vi "ProcessBotMove.vi"(7 "MatchState":T1, 8 "error in (no error)":errorcluster, 9 "GameState":T2, 10 "BotPosition":T3, 11 "Bot in":T4) -> (0 "error out":errorcluster, 2 "NewPlayerPosition":T3, 3 "Bot out":T4)   [LabVIEW 2015, in "TronviewGame.lvlib" / "Game.lvclass"]
uses:
  Game.lvclass
  BotVIRefnum.ctl
  Board/Position.ctl
  TronVIEWBotAPI/GameState.ctl
  TronVIEWBotAPI/MatchState.ctl
  Board/Board.lvclass
  TronVIEWBotAPI/TronVIEWBotAPI.lvlib
  TronviewGame.lvlib
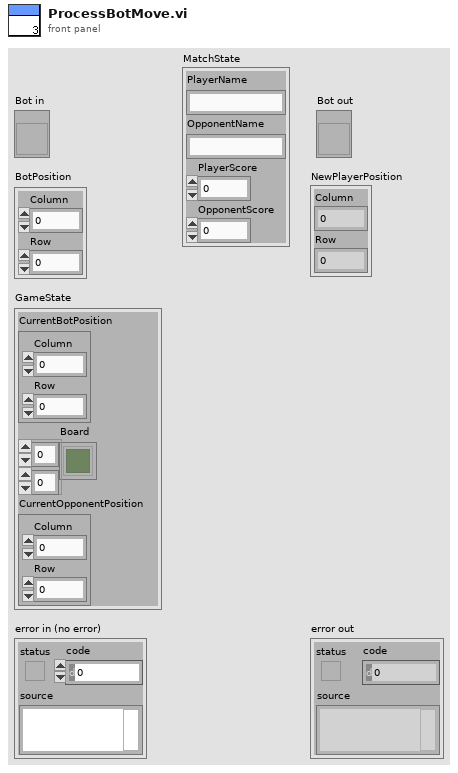
[diagram p1: front panel]
types:
  T1 = typedef "TronVIEWBotAPI.lvlib/MatchState.ctl" = cluster{"PlayerName":string, "OpponentName":string, "PlayerScore":u32, "OpponentScore":u32}
  T2 = typedef "TronVIEWBotAPI.lvlib/GameState.ctl" = cluster{"CurrentBotPosition":T3, "Board":bool[][], "CurrentOpponentPosition":T3}
  T3 = typedef "TronviewGame.lvlib/Board.lvclass/Position.ctl" = cluster{"Column":i32, "Row":i32}
  T4 = typedef "TronviewGame.lvlib/BotVIRefnum.ctl" = refnum<vi>
  T5 = typedef "TronVIEWBotAPI.lvlib/MovementDirection.ctl" = enum16{"N", "S", "W", "E"}
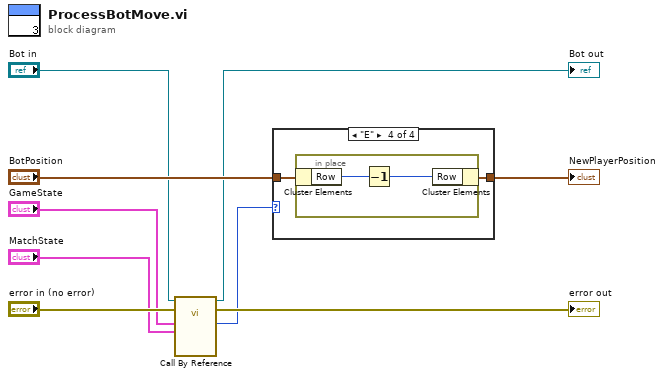
[diagram p0: block diagram]
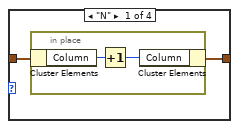
[diagram p2: hidden frame]
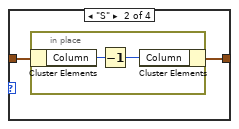
[diagram p3: hidden frame]
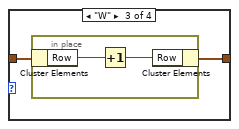
[diagram p4: hidden frame]
diagram:
  n1 = call-by-ref "?"(reference="Bot in", error in="error in (no error)", "MatchState"="MatchState", "GameState"="GameState") -> (reference out=→"Bot out":T4, error out=→"error out":errorcluster, "Move"=w3:T5)  [unwired: 9 in]
  n2 = case shown="\"E\"" w3 {
    tunnel: "BotPosition" -> [w11 w15 w19 w23]
    tunnel: [w10 w14 w18 w22] -> w8
    frame "N" {
      n3 = in-place {
        n4 = in-place-cluster #1(w11) -> ("Column"=w13:i32)
        n5 = Increment(x=w13) -> (x+1=w12:i32)
        n6 = in-place-cluster #1("Column"=w12) -> (w10:T3)
      }
    }
    frame "S" {
      n7 = in-place {
        n8 = in-place-cluster #2(w15) -> ("Column"=w17:i32)
        n9 = Decrement(x=w17) -> (x-1=w16:i32)
        n10 = in-place-cluster #2("Column"=w16) -> (w14:T3)
      }
    }
    frame "W" {
      n11 = in-place {
        n12 = in-place-cluster #3(w19) -> ("Row"=w21:i32)
        n13 = Increment(x=w21) -> (x+1=w20:i32)
        n14 = in-place-cluster #3("Row"=w20) -> (w18:T3)
      }
    }
    frame "E" {
      n15 = in-place {
        n16 = in-place-cluster #4(w23) -> ("Row"=w25:i32)
        n17 = Decrement(x=w25) -> (x-1=w24:i32)
        n18 = in-place-cluster #4("Row"=w24) -> (w22:T3)
      }
    }
  }
  "NewPlayerPosition" <- w8
